vi "Pockels-Mov Cor Ref scan cycles.vi"(11 "Imaging Protocol":T1) -> (3 "Ref Scan Cycles":i32)   [LabVIEW 2020]
uses:
  Typedefs/Imaging Protocols enum.ctl
  Globals/gl_Pockels control globals.vi
panel:
  # "<--- This is the time between reference frame triggers in FPGA clock cycles"
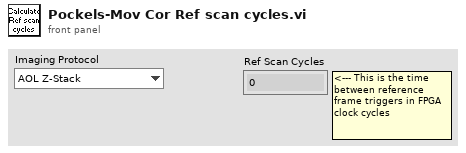
[diagram p1: front panel]
types:
  T1 = typedef "Imaging Protocols enum.ctl" = enum16{"AOL Z-Stack", "Motor Z Stack", "Functional Acquisition", "Single Plane Acquisition", "Volume Acquisition", "Live Imaging", "Live Plane Imaging", "Live Volume Imaging"}
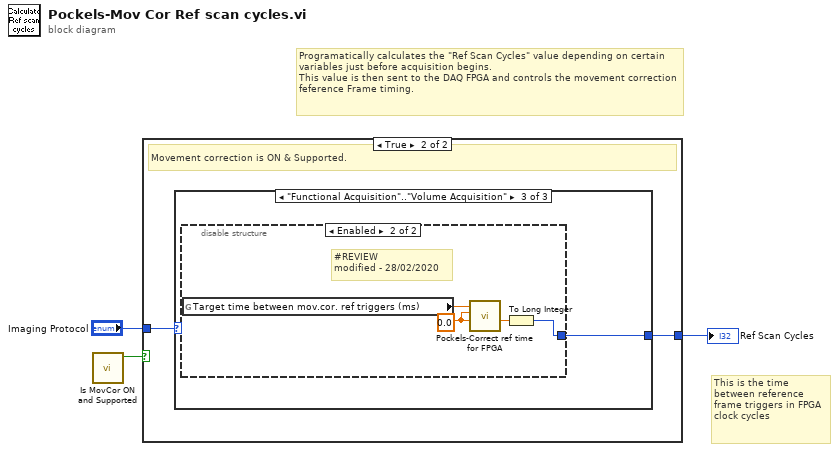
[diagram p0: block diagram]
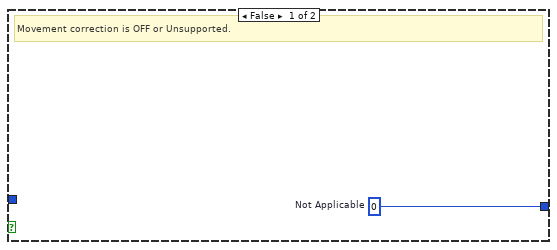
[diagram p2: hidden frame]
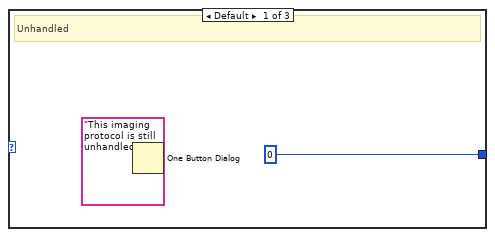
[diagram p3: hidden frame]
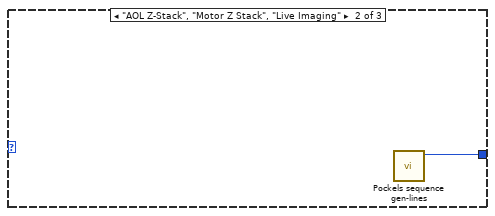
[diagram p4: hidden frame]
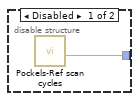
[diagram p5: hidden frame]
diagram:
  # "Programatically calculates the \"Ref Scan Cycles\" value depending on certain variables just before acquisition begins.\nThis value is then sent to the DAQ FPGA and controls the movement correction feference Frame timing."
  # "This is the time between reference frame triggers in FPGA clock cycles"
  n1 = call "Is MovCor ON and Supported.vi"() -> ("MovCor is ON and Supported"=w1:bool)  [unwired: 11 in]
  n2 = case shown="True" w1 {
    tunnel: [w4 w6] -> w3
    tunnel: "Imaging Protocol" -> [_ w5]
    frame False {
      w4 = 0  # Not Applicable
      # "Movement correction is OFF or Unsupported."
    }
    frame True {
      # "Movement correction is ON & Supported."
      n3 = case shown="\"Functional Acquisition\"..\"Volume Acquisition\"" w5 {
        tunnel: [0 ("Ref Scan Cycles") w9 w10] -> w6
        frame Default {
          # "Unhandled"
          n4 = One Button Dialog(message="This imaging protocol is still unhandled") -> ()  [unwired: 1 in, 1 out]
        }
        frame "AOL Z-Stack", "Motor Z Stack", "Live Imaging" {
          n5 = call "Pockels sequence gen-lines.vi"() -> ("Ref Scan Cycles"=w9:i32)  [unwired: 9 in, 2 out]
        }
        frame "Functional Acquisition".."Volume Acquisition" {
          n6 = disable-structure shown="Enabled" {
            disable-tunnel: [w11 w12] -> w10
            frame Disabled {
              n7 = call "Pockels-Ref scan cycles.vi"() -> ("Ref Scan Cycles"=w11:i32)  [unwired: 10 in, 1 out]
            }
            frame Enabled {
              w13 = 0.0 ("Time for main img line OR for a single POI (ms)")
              # "#REVIEW\nmodified - 28/02/2020"
              n8 = global read "gl_Pockels control globals.vi" "Target time between mov.cor. ref triggers (ms)"() -> (w15:dbl)
              n9 = call "Pockels-Correct ref time for FPGA.vi"("Fine tuning multiplier"=w13, "Time for main img line OR for a single POI (ms)"=w13, "Actual resulting time between ref triggers (ms)"=w15) -> ("Ref Scan Cycles"=w14:dbl)  [unwired: 7 in, 1 out]
              n10 = To Long Integer(number=w14) -> (32bit integer=w12:i32)
            }
          }
        }
      }
    }
  }
  "Ref Scan Cycles" <- w3
